vi "Set ServerReflection ServerReflectionInfo Response.vi"(7 "Streaming? (F)":bool, 8 "error in (no error)":errorcluster, 10 "Message Data":T1, 11 "gRPCid in":T3) -> (0 "error out":errorcluster)   [LabVIEW 2025, in "reflection_server.lvlib" / "ServerReflection.lvclass"]
uses:
  ServerReflection.lvclass
  <vilib>/gRPC/LabVIEW gRPC Library/Shared/grpcId.ctl
  ServerReflection.lvclass/ServerReflection.ctl
  reflection_server.lvlib
  <vilib>/gRPC/LabVIEW gRPC Library/grpc-lvsupport-release.lvlib
  RPC Messages/grpc_reflection_v1alpha_ServerReflectionRequest_message_request/grpc_reflection_v1alpha_ServerReflectionRequest_message_request.lvclass
  RPC Messages/grpc_reflection_v1alpha_ServerReflectionRequest.ctl
  RPC Messages/grpc_reflection_v1alpha_ServerReflectionResponse_message_response/grpc_reflection_v1alpha_ServerReflectionResponse_message_response.lvclass
  RPC Messages/grpc_reflection_v1alpha_ServerReflectionResponse.ctl
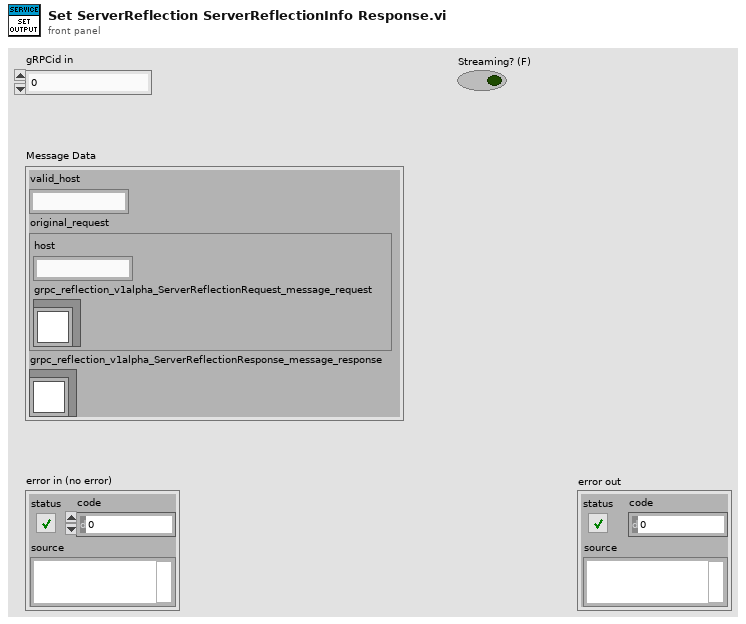
[diagram p1: front panel]
types:
  T1 = typedef "reflection_server.lvlib/grpc_reflection_v1alpha_ServerReflectionResponse.ctl" = cluster{"valid_host":string, "original_request":T2, "grpc_reflection_v1alpha_ServerReflectionResponse_message_response":refnum<class "grpc_reflection_v1alpha_ServerReflectionResponse_message_response.lvclass">}
  T2 = typedef "reflection_server.lvlib/grpc_reflection_v1alpha_ServerReflectionRequest.ctl" = cluster{"host":string, "grpc_reflection_v1alpha_ServerReflectionRequest_message_request":refnum<class "grpc_reflection_v1alpha_ServerReflectionRequest_message_request.lvclass">}
  T3 = typedef "grpc-lvsupport-release.lvlib/grpcId.ctl" = u64
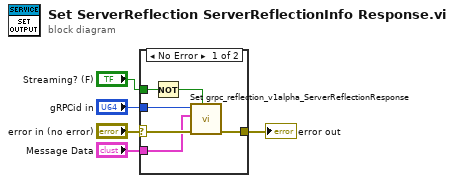
[diagram p0: block diagram]
diagram:
  n1 = case shown="No Error" "error in (no error)" {
    selector: "error in (no error)" -> [w11 w12]
    tunnel: [w9 w12] -> w4
    tunnel: "gRPCid in" -> [w10 _]
    tunnel: "Message Data" -> [w8 _]
    tunnel: "Streaming? (F)" -> [w7 _]
    frame No Error {
      n2 = Not(x=w7) -> (.not. x?=w6:bool)
      n3 = call "Set grpc_reflection_v1alpha_ServerReflectionResponse.vi"("Complete Call (T)"=w6, "error in (no error)"=w11, "package_templatemessage"=w8, "gRPCid"=w10) -> ("error out"=w9:errorcluster)  [unwired: 7 in]
    }
    frame Error {
    }
  }
  "error out" <- w4
